vi "Multi_Run_PostPro.vi"() -> ()   [LabVIEW 2017]
uses:
  Controls/saveDataOption.ctl
  Globals/measurementGlobal.vi
panel:
  out "Folder Path":path
  in  "No. Of Measurement Folders":i32=3
  in  "No. of Folders":i32=6
  in  "File Increment":dbl=0.2
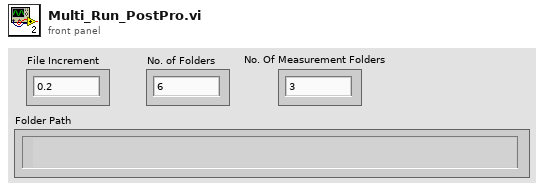
[diagram p1: front panel]
types:
  T1 = typedef "saveDataOption.ctl" = enum16{"Save Data", "Do Not Save Data"}
  T2 = enum16{"New Measurement", "Post-process Raw Data"}
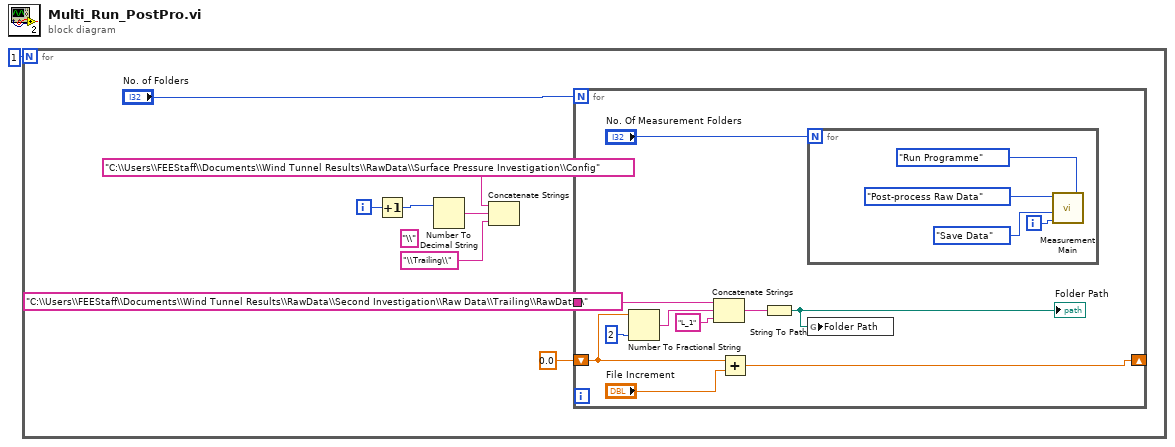
[diagram p0: block diagram]
diagram:
  n1 = for {
    N: 1 -> [_]
    i -> [w7]
    (unwired) "\\" ("string")
    n2 = Increment(x=w7) -> (x+1=w9:i32)
    n3 = Number To Decimal String(number=w9) -> (decimal integer string=w8:string)  [unwired: 1 in]
    n4 = Concatenate Strings("C:\\Users\\FEEStaff\\Documents\\Wind Tunnel Results\\RawData\\Surface Pressure Investigation\\Config", w8, "\\Trailing\\" ("string")) -> ()  [unwired: 1 out]
    n5 = for {
      N: "No. of Folders" -> [_]
      tunnel: "C:\\Users\\FEEStaff\\Documents\\Wind Tunnel Results\\RawData\\Second Investigation\\Raw Data\\Trailing\\RawData\\" -> [w15]
      shift-right: [w11] -> _
      shift-left: 0.0 -> [w13]
      n6 = Number To Fractional String(number=w13, precision (6)=i16 2) -> (F-format string=w19:string)  [unwired: 2 in]
      n7 = Concatenate Strings(w15, w19, "L_1" ("string")) -> (w14:string)
      n8 = Add(x=w13, y="File Increment") -> (x+y=w11:dbl)
      n9 = String To Path(string=w14) -> (path=w16:path)
      "Folder Path" <- w16
      n10 = for {
        N: "No. Of Measurement Folders" -> [_]
        i -> [w21]
        n11 = call "Measurement Main.vi"("Setup"=enum16{"Run Programme", "Show Setup"}."Run Programme", "No of Measurement File"=w21, "Save Data Option"=saveDataOption."Save Data", "Data Acquisition"=T2."Post-process Raw Data") -> ()  [unwired: 2 in]
      }
      n12 = global write "measurementGlobal.vi" "Folder Path"(w16) -> ()
    }
  }
